vi "Add Command_ex.vi"() -> ()   [LabVIEW 2019]
uses:
  <vilib>/NI VeriStand/Custom Device API/Custom Device Item Ref.ctl
  Control 5.ctl
  Control 15.ctl
  Scripting API/Scripting API.lvlib
  <vilib>/NI VeriStand/Custom Device API/Custom Device API.lvlib
panel:
  out "Message Refnum Out":T1=18446744073709551615 format="%.0x"
  out "Command Refnum":T1=18446744073709551615 format="%.0x"
  out "Error Out":errorcluster
  in  "Message Refnum In":T1=18446744073709551615 format="%.0x"
  in  "Error In":errorcluster
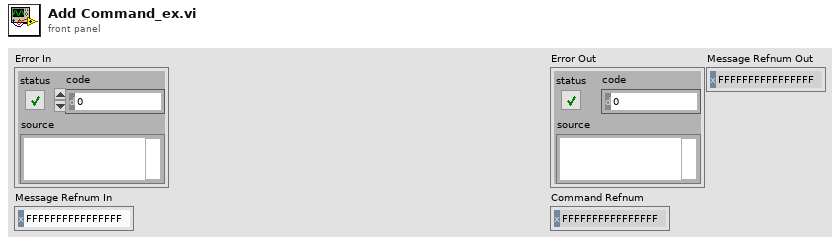
[diagram p1: front panel]
types:
  T1 = typedef "Custom Device API.lvlib/Custom Device Item Ref.ctl" = u64
  T2 = typedef "Control 5.ctl" = cluster{"Command Format":string, "Linkages":cluster{"Variable name":string, "Linked Channel refnum":T1}[], "Use Padding?":bool, "Padding":T3}
  T3 = typedef "Control 15.ctl" = cluster{"Length":u16, "Pad Value":u16}
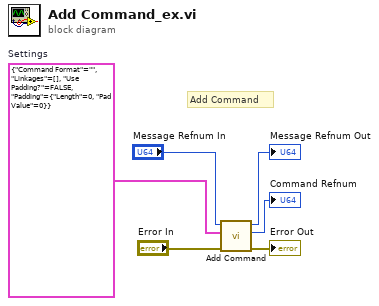
[diagram p0: block diagram]
diagram:
  w1 = T2 {"Command Format"="", "Linkages"=[], "Use Padding?"=FALSE, "Padding"={"Length"=0, "Pad Value"=0}}  # Settings
  # "Add Command"
  n1 = call "Add Command.vi"("Error In"="Error In", "Settings"=w1, "Message Refnum In"="Message Refnum In") -> ("Error Out"=→"Error Out":errorcluster, "Command Refnum"=→"Command Refnum":T1, "Message Refnum Out"=→"Message Refnum Out":T1)  [unwired: 6 in]
